vi "SCOPE Configuration_SA-Scope SP.vi"(6 "Timeout(10)":dbl=10.0, 7 "Operation":T1=enum."Initial", 8 "error in":errorcluster, 9 "Reset?(T)":bool=TRUE caption="reset device", 11 "Device. Name":string) -> (0 "error out":errorcluster, 1 "Status":string, 3 "InstruHandle":refnum<k15>, 4 "Rate":string, 5 "wfm":dbl[][](array[numeric]))   [LabVIEW 2012]
doc: "功能全局，处理对SCOPE的各种操作，包括：\n1.创建\n2.横向配置\n3.纵向配置\n4.触发配置\n5.关闭操作"
uses:
  <instrlib>/niScope/Controls/niScope vertical coupling.ctl
  <instrlib>/niScope/Controls/niScope self cal option.ctl
  Data Structure.llb/Function Variable Parameter Operations-Scope SP.ctl
  <instrlib>/niScope/Configure/Trigger/niScope Configure Trigger Window.vi
  <instrlib>/niScope/Configure/Trigger/niScope Configure Trigger Digital.vi
  <instrlib>/niScope/Configure/Trigger/niScope Configure Trigger Immediate.vi
  <instrlib>/niScope/Configure/Trigger/niScope Configure Trigger Hysteresis.vi
  <instrlib>/niScope/Configure/Trigger/niScope Configure Video Trigger.vi
  <instrlib>/niScope/Configure/Trigger/niScope Configure Trigger Edge.vi
  <instrlib>/niScope/Acquire/Fetch/niScope Multi Fetch.vi
  <instrlib>/niScope/Acquire/Fetch/niScope Fetch.vi
  <instrlib>/niScope/Configure/Trigger/niScope Configure Trigger Software.vi
  <instrlib>/NISCOPE/Controls/niScope scalar measurement.ctl
  SCOPE Operations_SA-Scope SP.ctl
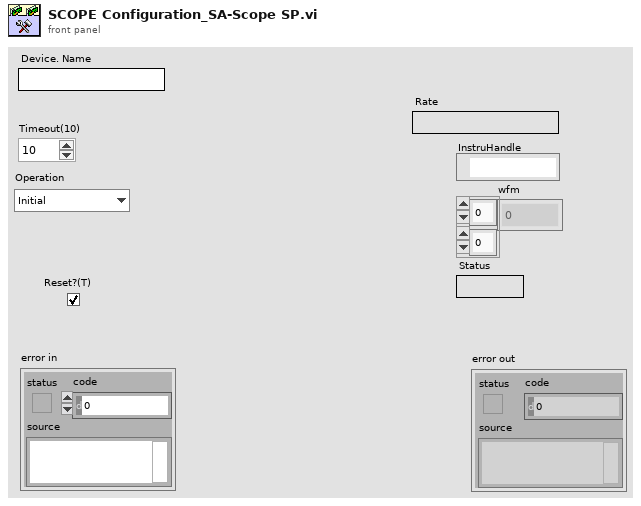
[diagram p1: front panel]
types:
  T1 = typedef "SCOPE Operations_SA-Scope SP.ctl" = enum16{"Noop", "Initial", "Horizontal", "Vertical", "Trigger", "RIS", "Initiate", "Fetch", "Abort", "Close", "SelfCalibrate", "AutoSetup"}
  T2 = typedef "Function Variable Parameter Operations-Scope SP.ctl" = enum16{"Set", "Get"}
  T3 = typedef "INI Initial Values_DStr-Scope SP.ctl" = cluster{"Active0":i32, "Acitive1":i32, "Channel":i32[], "ChanEnable":bool[], "ChanCpl":i32[], "OffsetVisible":bool[], "Offset":dbl[], "VoltInterval":i32[], "ProbAttenu":i32[], "Impedance":i32[], "BandWidth":i32[], "VertiPosi":dbl[], "Range":dbl[], "TimeInterval":i32, "Points":i32, "RefPosition":dbl, "Type":i32, "Source":i32, "TrigCpl":i32, "ExtCpl":i32, "Mode":i32, "Slope":i32, "Level":dbl, "Hyster":dbl, "WinMode":i32, "WinLow":dbl, "WinHigh":dbl, "Polarity":i32, "Event":i32, "Format":i32, "Line":i32, "DCRestore":bool, "RIS":bool, "Rate":dbl, "DigiSource":i32}
  T4 = typedef "INI Properties_DStr-Scope SP.ctl" = cluster{"Channels":cluster{"String":string, "Value":ext}[], "VoltInterval":cluster{"String":string, "Value":ext}[], "Impedance":cluster{"String":string, "Value":ext}[], "Bandwidth":cluster{"String":string, "Value":ext}[], "TimeInterval":cluster{"String":string, "Value":ext}[], "Type":cluster{"String":string, "Value":ext}[], "Source":cluster{"String":string, "Value":ext}[], "DigiSource":cluster{"String":string, "Value":ext}[], "TrigCpl":cluster{"String":string, "Value":ext}[], "EXTCpl":cluster{"String":string, "Value":ext}[], "Mode":cluster{"String":string, "Value":ext}[], "Event":cluster{"String":string, "Value":ext}[], "Format":cluster{"String":string, "Value":ext}[], "OffsetVisible":bool[], "Offset":dbl[][], "Point":dbl[][], "TrigLev":dbl[][], "Win":dbl[][], "Leve":dbl[][], "ExtLev":dbl[][], "PolaEnable":u8, "RISEnable":u8, "ChanCpl":cluster{"String":string, "Value":ext}[], "TimeValue":dbl[], "VoltValue":dbl[], "ImpedanceValue":dbl[], "BandwidthValue":dbl[]}
  T5 = typedef "niScope scalar measurement.ctl" = i32
  T6 = typedef "niScope vertical coupling.ctl" = i32
  T7 = cluster{"actualSamples":i32, "absoluteInitialX":dbl, "relativeInitialX":dbl, "xIncrement":dbl, "offset":dbl, "gain":dbl, "reserved1":dbl, "reserved2":dbl}
  T8 = cluster{"actualSamples":i32, "absoluteInitialX":dbl, "relativeInitialX":dbl, "xIncrement":dbl, "offset":dbl, "gain":dbl, "reserved1":dbl, "reserved2":dbl}[]
  T9 = typedef "niScope self cal option.ctl" = i32
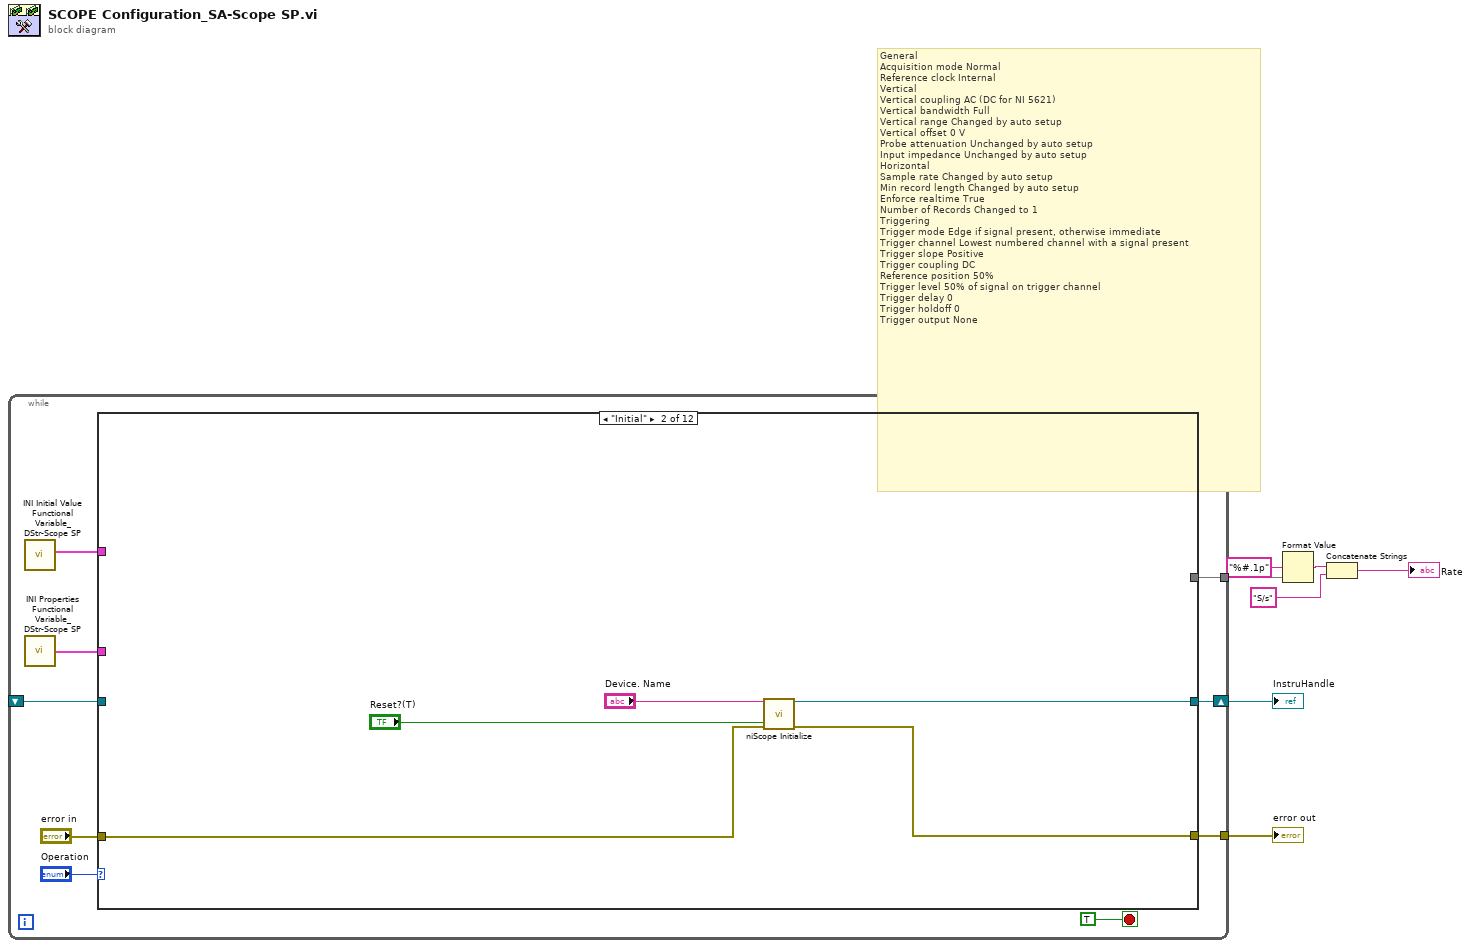
[diagram p0: block diagram]
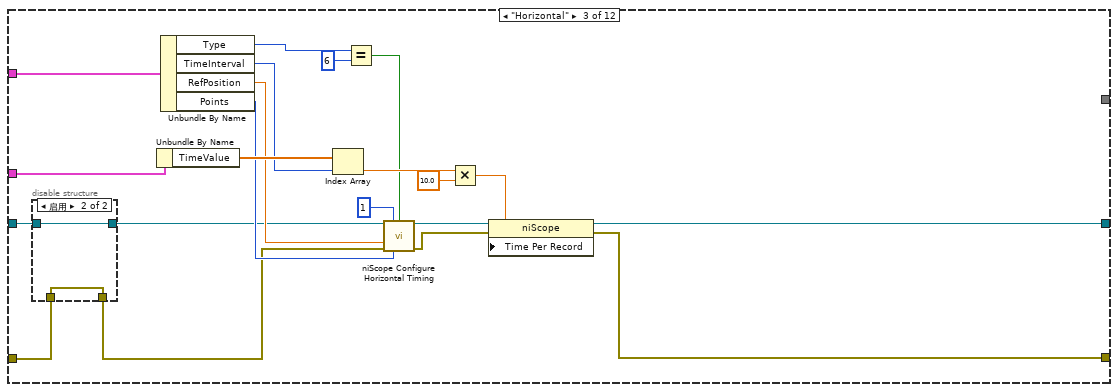
[diagram p3: hidden frame]
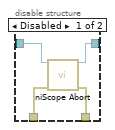
[diagram p4: hidden frame]
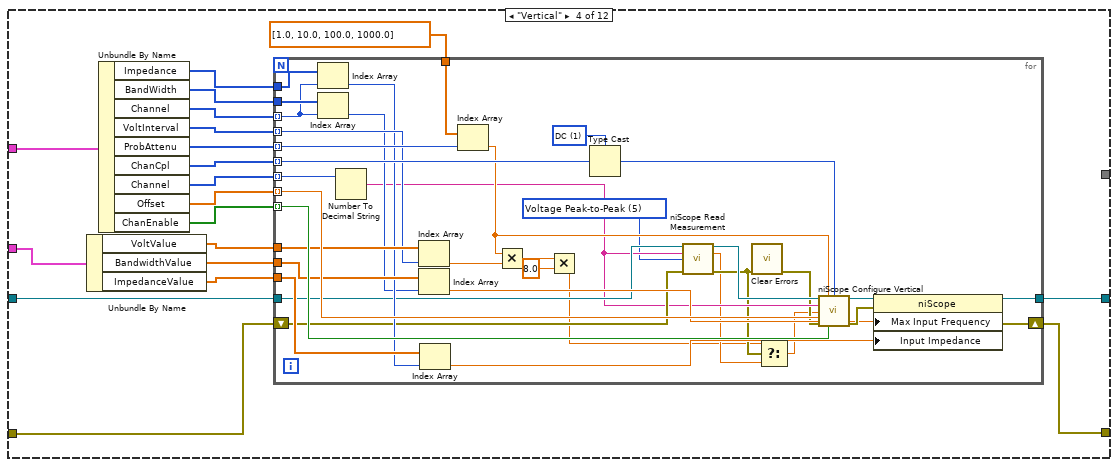
[diagram p5: hidden frame]
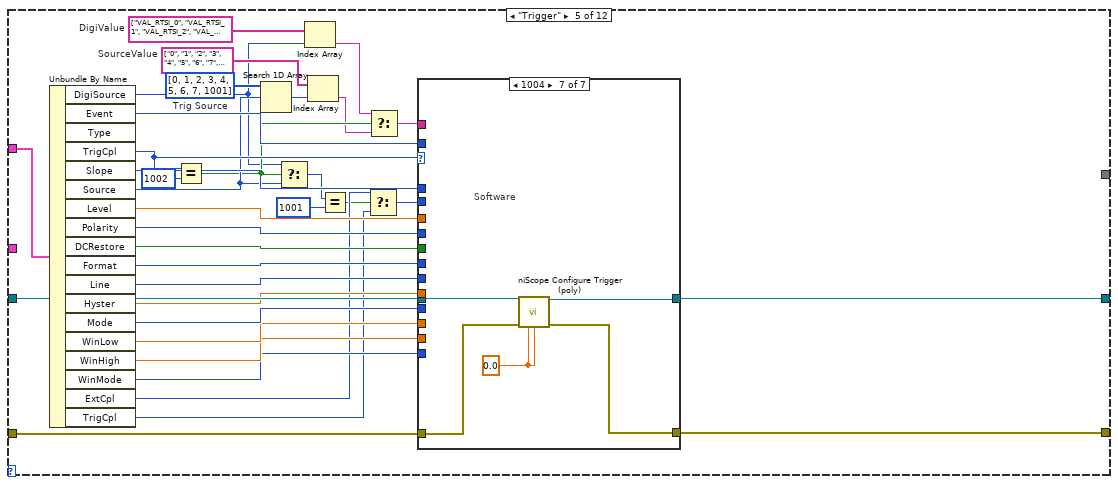
[diagram p6: hidden frame]
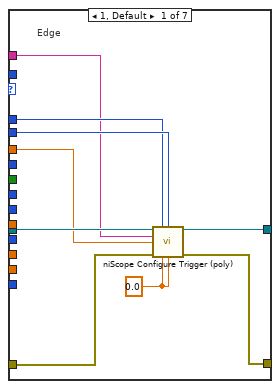
[diagram p7: hidden frame]
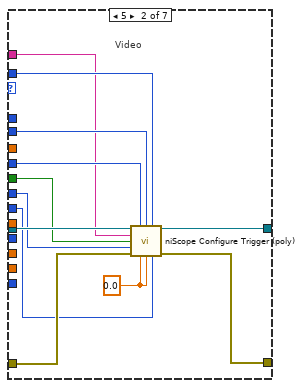
[diagram p8: hidden frame]
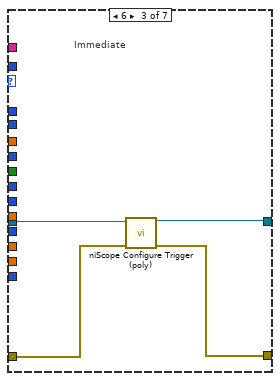
[diagram p9: hidden frame]
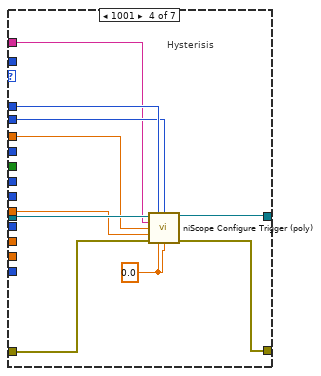
[diagram p10: hidden frame]
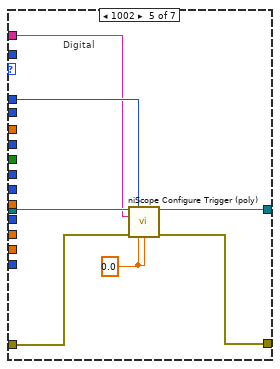
[diagram p11: hidden frame]
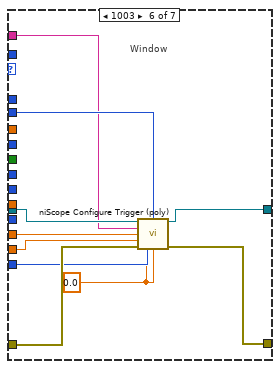
[diagram p12: hidden frame]
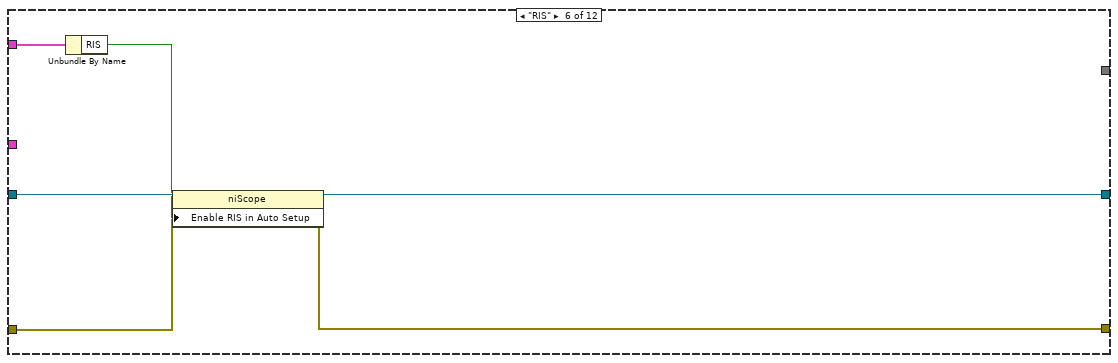
[diagram p13: hidden frame]
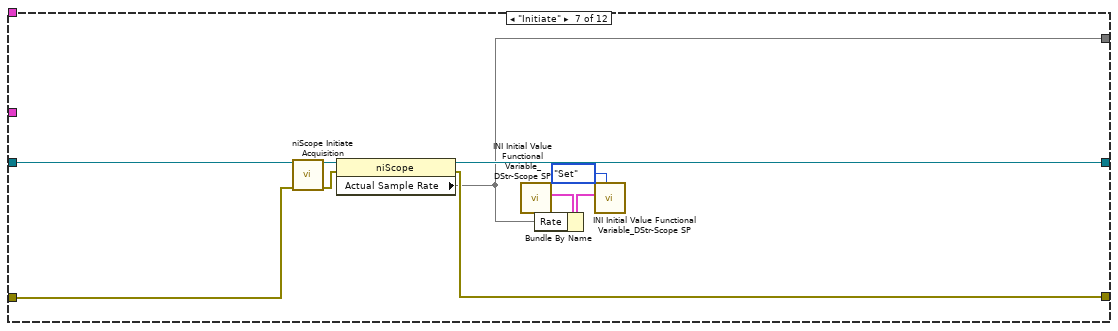
[diagram p14: hidden frame]
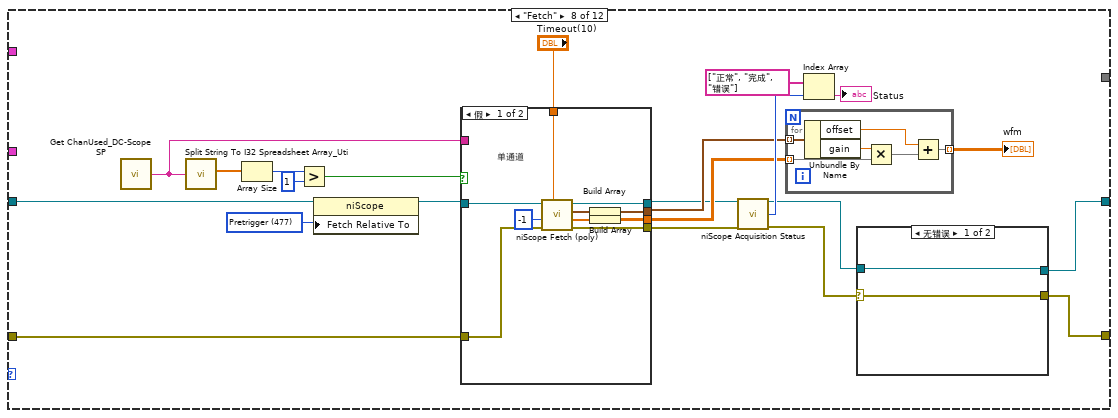
[diagram p15: hidden frame]
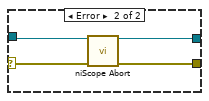
[diagram p16: hidden frame]
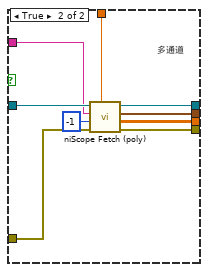
[diagram p17: hidden frame]
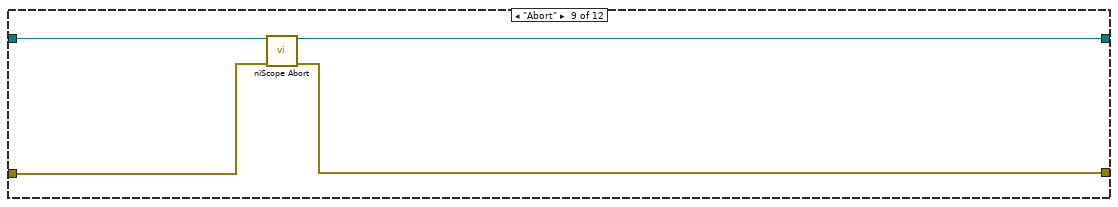
[diagram p18: hidden frame]
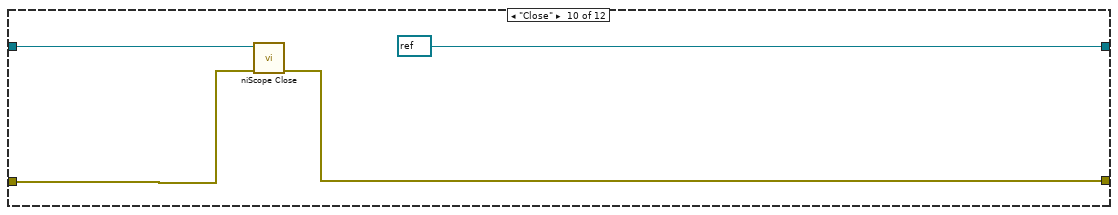
[diagram p19: hidden frame]
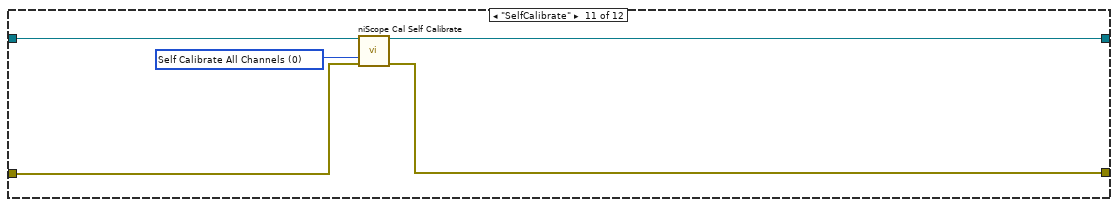
[diagram p20: hidden frame]
diagram:
  # "General \nAcquisition mode Normal  \nReference clock Internal  \nVertical \nVertical coupling AC (DC for NI 5621)  \nVertical bandwidth Full  \nVertical range Changed by auto setup  \nVertical offset 0 V  \nProbe attenuation Unchanged by auto setup  \nInput impedance Unchanged by auto setup  \nHorizontal \nSample rate Changed by auto setup  \nMin record length Changed by auto setup  \nEnforce realtime True  \nNumber of Records Changed to 1 \nTriggering \nTrigger mode Edge if signal present, otherwise immediate  \nTrigger channel Lowest numbered channel with a signal present  \nTrigger slope Positive  \nTrigger coupling DC  \nReference position 50%  \nTrigger level 50% of signal on trigger channel  \nTrigger delay 0  \nTrigger holdoff 0  \nTrigger output None"
  n1 = while {
    shift-right: [w14] -> w6
    shift-left: _ -> [w11]
    tunnel: [w12] -> w7
    tunnel: [w8] -> w2
    stop <- TRUE stop-if-true
    n2 = call "INI Initial Value Functional Variable_DStr-Scope SP.vi"() -> ("Value out"=w10:T3)  [unwired: 10 in, 1 out]
    n3 = call "INI Properties Functional Variable_DStr-Scope SP.vi"() -> ("proper"=w9:T4)  [unwired: 15 in]
    n4 = case shown="\"Initial\"" "Operation" {
      tunnel: [w18 w20 w41 w66 w139 w199 w209 w215 w268 refnum<k15> refnum ("instrument handle out") w277 w284] -> w14
      tunnel: "error in" -> [w17 w23 w27 w68 w141 w201 w213 w226 w270 w274 w279 w308]
      tunnel: [w17 w19 w38 w67 w140 w200 w208 w217 w269 w273 w278 w293] -> w12
      tunnel: w11 -> [w18 _ w26 w69 w138 w204 w214 w227 w271 w275 w280 w309]
      tunnel: w10 -> [_ _ w44 w65 w137 w203 _ _ _ _ _ w301]
      tunnel: w9 -> [_ _ w34 w58 _ _ _ _ _ _ _ w292]
      tunnel: [_ _ _ _ _ _ w207 _ _ _ _ w287] -> w8
      frame "Noop", Default {
      }
      frame "Initial" {
        n5 = call <instrlib>:"niScope Initialize.vi"("resource name"="Device. Name", "reset device"="Reset?(T)", "error in"=w23) -> ("instrument handle"=w20:refnum<k15>, "error out"=w19:errorcluster)  [unwired: 11 in]
      }
      frame "Horizontal" {
        n6 = disable-structure shown="启用" {
          disable-tunnel: w27 -> [w48 w49]
          disable-tunnel: w26 -> [w47 w50]
          disable-tunnel: [w46 w50] -> w25
          disable-tunnel: [w45 w49] -> w24
          frame Disabled {
            n7 = call <instrlib>:"niScope Abort.vi"("instrument handle"=w47, "error in"=w48) -> ("instrument handle out"=w46:refnum<k15>, "error out"=w45:errorcluster)  [unwired: 12 in]
          }
          frame Enabled {
          }
        }
        n8 = Unbundle By Name(w34) -> ("TimeValue"=w40:dbl[])
        n9 = Unbundle By Name(w44) -> ("Type"=w33:i32, "TimeInterval"=w30:i32, "RefPosition"=w28:dbl, "Points"=w29:i32)
        n10 = Index Array(array=w40, index=w30) -> (element=w37:dbl)
        n11 = Equal?(x=w33, y=6) -> (x = y?=w31:bool)
        n12 = call <instrlib>:"niScope Configure Horizontal Timing.vi"("instrument handle"=w25, "number of records"=1 ("f"), "enforce realtime"=w31, "reference position"=w28, "error in"=w24, "min record length"=w29) -> ("instrument handle out"=w42:refnum<k15>, "error out"=w39:errorcluster)  [unwired: 8 in]
        n13 = Multiply(x=w37, y=10.0) -> (x*y=w35:dbl)
        n14 = property class="niScope"(reference=w42, error in=w39, "Time Per Record"=w35) -> (reference out=w41:refnum<k15>, error out=w38:errorcluster)
      }
      frame "Vertical" {
        n15 = Unbundle By Name(w58) -> ("VoltValue"=w57:dbl[], "BandwidthValue"=w55:dbl[], "ImpedanceValue"=w54:dbl[])
        n16 = Unbundle By Name(w65) -> ("Impedance"=w52:i32[], "BandWidth"=w51:i32[], "Channel"=w53:i32[], "VoltInterval"=w56:i32[], "ProbAttenu"=w64:i32[], "ChanCpl"=w62:i32[], "Channel"=w61:i32[], "Offset"=w60:dbl[], "ChanEnable"=w59:bool[])
        n17 = for {
          tunnel: w69 -> [w78]
          shift-right: [w91] -> w67
          shift-left: w68 -> [w79]
          tunnel: [w93] -> w66
          tunnel: w64 -> [w99] mode=indexing
          tunnel: dbl[] [1.0, 10.0, 100.0, 1000.0] -> [w104]
          tunnel: w62 -> [w100] mode=indexing
          tunnel: w61 -> [w103] mode=indexing
          tunnel: w60 -> [w102] mode=indexing
          tunnel: w59 -> [w101] mode=indexing
          tunnel: w57 -> [w98]
          tunnel: w56 -> [w88] mode=indexing
          tunnel: w55 -> [w90]
          tunnel: w54 -> [w89]
          tunnel: w53 -> [w82] mode=indexing
          tunnel: w52 -> [w84]
          tunnel: w51 -> [w83]
          w75 = T5 5 items=["None"=4000, "Frequency"=2, "Average Frequency"=1016, "FFT Frequency"=1008, "Period"=3, "Average Period"=1015, "Rise Time"=0, "Fall Time"=1, "Rising Slew Rate"=1010, "Falling Slew Rate"=1011, "Overshoot"=18, "Preshoot"=19, "Voltage RMS"=4, "Voltage Cycle RMS"=16, "AC Estimate"=1012, "FFT Amplitude"=1009, "Voltage Average"=10, "Voltage Cycle Average"=17, "DC Estimate"=1013, "Voltage Max"=6, "Voltage Min"=7, "Voltage Peak-to-Peak"=5, "Voltage High"=8, "Voltage Low"=9, "Voltage Amplitude"=15, "Voltage Top"=1007, "Voltage Base"=1006, "Voltage Base-to-Top"=1017, "Negative Width"=11, "Positive Width"=12, "Negative Duty Cycle"=13, "Positive Duty Cycle"=14, "Integral"=1005, "Area"=1003, "Cycle Area"=1004, "Time Delay"=1014, "Phase Delay"=1018, "Low Ref Volts"=1000, "Mid Ref Volts"=1001, "High Ref Volts"=1002, "Volt. Hist. Mean"=2000, "Volt. Hist. Stdev"=2001, "Volt. Hist. Median"=2003, "Volt. Hist. Mode"=2010, "Volt. Hist. Max"=2005, "Volt. Hist. Min"=2006, "Volt. Hist. Peak-to-Peak"=2002, "Volt. Hist. Mean + Stdev"=2007, "Volt. Hist. Mean + 2 Stdev"=2008, "Volt. Hist. Mean + 3 Stdev"=2009, "Volt. Hist. Hits"=2004, "Volt. Hist. New Hits"=2011, "Time Hist. Mean"=3000, "Time Hist. Stdev"=3001, "Time Hist. Median"=3003, "Time Hist. Mode"=3010, "Time Hist. Max"=3005, "Time Hist. Min"=3006, "Time Hist. Peak-to-Peak"=3002, "Time Hist. Mean + Stdev"=3007, "Time Hist. Mean + 2 Stdev"=3008, "Time Hist. Mean + 3 Stdev"=3009, "Time Hist. Hits"=3004, "Time Hist. New Hits"=3011] ("scalar measurement")
          w106 = T6 1 items=["AC", "DC", "Ground"] ("vertical coupling")
          n18 = Index Array(array=w84, index=w82) -> (element=w81:i32)
          n19 = Index Array(array=w83, index=w82) -> (element=w80:i32)
          n20 = Number To Decimal String(number=w103) -> (decimal integer string=w76:string)  [unwired: 1 in]
          n21 = Index Array(array=w98, index=w88) -> (element=w97:dbl)
          n22 = Index Array(array=w90, index=w80) -> (element=w87:dbl)
          n23 = Index Array(array=w89, index=w81) -> (element=w86:dbl)
          n24 = Index Array(array=w104, index=w99) -> (element=w96:dbl)
          n25 = Multiply(x=w96, y=w97) -> (x*y=w95:dbl)
          n26 = Multiply(x=w95, y=8.0) -> (x*y=w70:dbl)
          n27 = Type Cast(type=w106, x=w100) -> (*(type *) &x=w105:T6)
          n28 = call <instrlib>:"niScope Read Measurement.vi"("instrument handle"=w78, "channels"=w76, "scalar measurement"=w75, "error in"=w79) -> ("instrument handle out"=w77:refnum<k15>, "result"=w71:dbl, "error out"=w73:errorcluster)  [unwired: 9 in]
          n29 = call <vilib>:"Clear Errors.vi"("error in (no error)"=w73) -> ("error out"=w74:errorcluster)  [unwired: 6 in]
          n30 = Select(t=w70, s=w73, f=w71) -> (s? t:f=w72:dbl)
          n31 = call <instrlib>:"niScope Configure Vertical.vi"("instrument handle"=w77, "probe attenuation"=w96, "vertical coupling"=w105, "channels"=w76, "vertical range"=w72, "vertical offset"=w102, "error in"=w74, "channel enabled"=w101) -> ("instrument handle out"=w94:refnum<k15>, "error out"=w92:errorcluster)  [unwired: 6 in]
          n32 = property class="niScope"(reference=w94, error in=w92, "Max Input Frequency"=w87, "Input Impedance"=w86) -> (reference out=w93:refnum<k15>, error out=w91:errorcluster)
        }
      }
      frame "Trigger" {
        w110 = string[] ["VAL_RTSI_0", "VAL_RTSI_1", "VAL_RTSI_2", "VAL_RTSI_3", "VAL_RTSI_4", "VAL_RTSI_5", "VAL_RTSI_6", "VAL_PFI_0", "VAL_PFI_1", "VAL_PFI_2", "VAL_PXI_STAR"]  # DigiValue
        w116 = string[] ["0", "1", "2", "3", "4", "5", "6", "7", "VAL_EXTERNAL"]  # SourceValue
        w114 = i32[] [0, 1, 2, 3, 4, 5, 6, 7, 1001]  # Trig Source
        n33 = Unbundle By Name(w137) -> ("DigiSource"=w109:i32, "Event"=w134:i32, "Type"=w121:i32, "Slope"=w136:i32, "Source"=w113:i32, "Level"=w135:dbl, "Polarity"=w133:i32, "DCRestore"=w132:bool, "Format"=w131:i32, "Line"=w130:i32, "Hyster"=w129:dbl, "Mode"=w128:i32, "WinLow"=w127:dbl, "WinHigh"=w126:dbl, "WinMode"=w125:i32, "ExtCpl"=w124:i32, "TrigCpl"=w122:i32)  [unwired: 1 out]
        n34 = Equal?(x=w121, y=1002) -> (x = y?=w112:bool)
        n35 = Search 1D Array(1D array=w114, element=w113) -> (index of element=w115:i32)  [unwired: 1 in]
        n36 = Select(t=w109, s=w112, f=w113) -> (s? t:f=w119:i32)
        n37 = Index Array(array=w110, index=w109) -> (element=w108:string)
        n38 = Index Array(array=w116, index=w115) -> (element=w111:string)
        n39 = Equal?(x=w119, y=1001) -> (x = y?=w117:bool)
        n40 = Select(t=w124, s=w117, f=w122) -> (s? t:f=w123:i32)
        n41 = Select(t=w108, s=w112, f=w111) -> (s? t:f=w107:string)
        n42 = case shown="1004" w121 {
          tunnel: w138 -> [w150 w162 w166 w176 w183 w193 w198]
          tunnel: [w143 w160 w164 w174 w181 w191 w196] -> w139
          tunnel: w141 -> [w149 w161 w165 w175 w182 w192 w197]
          tunnel: [w142 w159 w163 w173 w180 w190 w195] -> w140
          tunnel: w123 -> [w147 w158 _ w170 _ w189 _]
          tunnel: w136 -> [w146 _ _ w172 w179 _ _]
          tunnel: w135 -> [w148 _ _ w171 _ _ _]
          tunnel: w134 -> [_ w157 _ _ _ _ _]
          tunnel: w133 -> [_ w156 _ _ _ _ _]
          tunnel: w107 -> [w144 w155 _ w169 w178 w188 _]
          tunnel: w132 -> [_ w154 _ _ _ _ _]
          tunnel: w131 -> [_ w153 _ _ _ _ _]
          tunnel: w130 -> [_ w151 _ _ _ _ _]
          tunnel: w129 -> [_ _ _ w168 _ _ _]
          tunnel: w128 -> [_ _ _ _ _ _ _]
          tunnel: w127 -> [_ _ _ _ _ w187 _]
          tunnel: w126 -> [_ _ _ _ _ w186 _]
          tunnel: w125 -> [_ _ _ _ _ w185 _]
          frame 1, Default {
            w145 = 0.0 ("trigger holdoff")
            # "Edge"
            n43 = call-poly <instrlib>:"niScope Configure Trigger (poly).vi"("instrument handle"=w150, "trigger slope"=w146, "trigger coupling"=w147, "trigger source"=w144, "trigger level"=w148, "error in"=w149, "trigger holdoff"=w145, "trigger delay"=w145) -> ("instrument handle out"=w143:refnum<k15>, "error out"=w142:errorcluster)  [unwired: 6 in]
          }
          frame 5 {
            w152 = 0.0 ("trigger holdoff")
            # "Video"
            n44 = call-poly <instrlib>:"niScope Configure Trigger (poly).vi"("instrument handle"=w162, "polarity"=w156, "trigger coupling"=w158, "TV event"=w157, "trigger source"=w155, "enable DC restore"=w154, "signal format"=w153, "error in"=w161, "trigger holdoff"=w152, "trigger delay"=w152, "line number"=w151) -> ("instrument handle out"=w160:refnum<k15>, "error out"=w159:errorcluster)  [unwired: 3 in]
          }
          frame 6 {
            # "Immediate"
            n45 = call-poly <instrlib>:"niScope Configure Trigger (poly).vi"("instrument handle"=w166, "error in"=w165) -> ("instrument handle out"=w164:refnum<k15>, "error out"=w163:errorcluster)  [unwired: 12 in]
          }
          frame 1001 {
            w167 = 0.0 ("trigger holdoff")
            # "Hysterisis"
            n46 = call-poly <instrlib>:"niScope Configure Trigger (poly).vi"("instrument handle"=w176, "trigger slope"=w172, "trigger coupling"=w170, "trigger source"=w169, "trigger level"=w171, "hysteresis"=w168, "error in"=w175, "trigger holdoff"=w167, "trigger delay"=w167) -> ("instrument handle out"=w174:refnum<k15>, "error out"=w173:errorcluster)  [unwired: 5 in]
          }
          frame 1002 {
            w177 = 0.0 ("trigger holdoff")
            # "Digital"
            n47 = call-poly <instrlib>:"niScope Configure Trigger (poly).vi"("instrument handle"=w183, "trigger slope"=w179, "trigger source"=w178, "error in"=w182, "trigger holdoff"=w177, "trigger delay"=w177) -> ("instrument handle out"=w181:refnum<k15>, "error out"=w180:errorcluster)  [unwired: 8 in]
          }
          frame 1003 {
            w184 = 0.0 ("trigger delay")
            # "Window"
            n48 = call-poly <instrlib>:"niScope Configure Trigger (poly).vi"("instrument handle"=w193, "trigger window mode"=w185, "trigger coupling"=w189, "trigger source"=w188, "low level"=w187, "high level"=w186, "error in"=w192, "trigger holdoff"=w184, "trigger delay"=w184) -> ("instrument handle out"=w191:refnum<k15>, "error out"=w190:errorcluster)  [unwired: 5 in]
          }
          frame 1004 {
            w194 = 0.0 ("trigger holdoff")
            # "Software"
            n49 = call-poly <instrlib>:"niScope Configure Trigger (poly).vi"("instrument handle"=w198, "error in"=w197, "trigger holdoff"=w194, "trigger delay"=w194) -> ("instrument handle out"=w196:refnum<k15>, "error out"=w195:errorcluster)  [unwired: 10 in]
          }
        }
      }
      frame "RIS" {
        n50 = Unbundle By Name(w203) -> ("RIS"=w202:bool)
        n51 = property class="niScope"(reference=w204, error in=w201, "Enable RIS in Auto Setup"=w202) -> (reference out=w199:refnum<k15>, error out=w200:errorcluster)
      }
      frame "Initiate" {
        n52 = call <instrlib>:"niScope Initiate Acquisition.vi"("instrument handle"=w214, "error in"=w213) -> ("instrument handle out"=w206:refnum<k15>, "error out"=w205:errorcluster)  [unwired: 12 in]
        n53 = property class="niScope"(reference=w206, error in=w205) -> (reference out=w209:refnum<k15>, error out=w208:errorcluster, "Actual Sample Rate"=w207)
        n54 = call "INI Initial Value Functional Variable_DStr-Scope SP.vi"() -> ("Value out"=w212:T3)  [unwired: 10 in, 1 out]
        n55 = Bundle By Name(cluster=w212, "Rate"=w207) -> (w211:T3)
        n56 = call "INI Initial Value Functional Variable_DStr-Scope SP.vi"("Mode(Get)"=Function_Variable_Parameter_Operations-Scope_SP."Set", "Value in"=w211) -> ()  [unwired: 8 in, 2 out]
      }
      frame "Fetch" {
        w221 = 477 items=["Start"=482, "Trigger"=483, "Pretrigger"=477, "Now"=481, "Read Pointer"=388] ("Fetch:Fetch Relative To")
        n57 = call "Get ChanUsed_DC-Scope SP.vi"() -> ("ChanUsed"=w219:string)  [unwired: 1 in]
        n58 = call "Split String To I32 Spreadsheet Array_Uti.vi"("StringIn"=w219) -> ("Array"=w236:dbl[])  [unwired: 8 in, 1 out]
        n59 = Array Size(array=w236) -> (size(s)=w235:i32)
        n60 = Greater?(x=w235, y=1) -> (0:w233:bool)
        n61 = property class="niScope"(reference=w227, "Fetch Relative To"=w221) -> (reference out=w222:refnum<k15>)  [unwired: 1 in, 1 out]
        n62 = case shown="假" w233 {
          tunnel: w222 -> [w258 w267]
          tunnel: w226 -> [w257 w266]
          tunnel: [w256 w265] -> w231
          tunnel: [w255 w264] -> w223
          tunnel: [w251 w261] -> w225
          tunnel: [w250 w262] -> w224
          tunnel: "Timeout(10)" -> [w252 w263]
          tunnel: w219 -> [_ w259]
          frame False {
            # "单通道"
            n63 = call-poly <instrlib>:"niScope Fetch (poly).vi"("timeout"=w252, "error in"=w257, "numSamples"=-1, "instrument handle"=w258) -> ("error out"=w256:errorcluster, "wfm"=w253:dbl[], "wfm info"=w254:T7, "instrument handle out"=w255:refnum<k15>)  [unwired: 4 in]
            n64 = Build Array(w254) -> (w251:T8)
            n65 = Build Array(w253) -> (w250:dbl[][])
          }
          frame True {
            # "多通道"
            n66 = call-poly <instrlib>:"niScope Fetch (poly).vi"("timeout"=w263, "error in"=w266, "numSamples"=-1, "channels"=w259, "instrument handle"=w267) -> ("error out"=w265:errorcluster, "wfm"=w262:dbl[][], "wfm info"=w261:T8, "instrument handle out"=w264:refnum<k15>)  [unwired: 3 in]
          }
        }
        n67 = call <instrlib>:"niScope Acquisition Status.vi"("instrument handle"=w223, "error in"=w231) -> ("instrument handle out"=w216:refnum<k15>, "acquisition status"=w228:i32, "error out"=w218:errorcluster)  [unwired: 11 in]
        n68 = for {
          tunnel: w225 -> [w248] mode=indexing
          tunnel: w224 -> [w246] mode=indexing
          tunnel: [w243] -> w220 mode=indexing
          n69 = Unbundle By Name(w248) -> ("offset"=w244:dbl, "gain"=w247:dbl)
          n70 = Multiply(x=w247, y=w246) -> (x*y=w245:dbl[])
          n71 = Add(x=w244, y=w245) -> (x+y=w243:dbl[])
        }
        "wfm" <- w220
        n72 = Index Array(array=string[] ["正常", "完成", "错误"], index=w228) -> (element=→"Status":string)
        n73 = case shown="无错误" w218 {
          selector: w218 -> [w238 w242]
          tunnel: [w238 w241] -> w217
          tunnel: w216 -> [w237 w240]
          tunnel: [w237 w239] -> w215
          frame No Error {
          }
          frame Error {
            n74 = call <instrlib>:"niScope Abort.vi"("instrument handle"=w240, "error in"=w242) -> ("instrument handle out"=w239:refnum<k15>, "error out"=w241:errorcluster)  [unwired: 12 in]
          }
        }
      }
      frame "Abort" {
        n75 = call <instrlib>:"niScope Abort.vi"("instrument handle"=w271, "error in"=w270) -> ("instrument handle out"=w268:refnum<k15>, "error out"=w269:errorcluster)  [unwired: 12 in]
      }
      frame "Close" {
        n76 = call <instrlib>:"niScope Close.vi"("instrument handle"=w275, "error in"=w274) -> ("error out"=w273:errorcluster)  [unwired: 13 in]
      }
      frame "SelfCalibrate" {
        w276 = T9 0 items=["Self Calibrate All Channels", "Restore External Calibration"] ("Option")
        n77 = call <instrlib>:"niScope Cal Self Calibrate.vi"("instrument handle"=w280, "Option"=w276, "error in"=w279) -> ("instrument handle out"=w277:refnum<k15>, "error out"=w278:errorcluster)  [unwired: 11 in]
      }
      frame "AutoSetup" {
        n78 = Unbundle By Name(w301) -> ("Channel"=w303:i32[], "VoltInterval"=w282:i32[])
        n79 = Unbundle By Name(w292) -> ("TimeValue"=w291:dbl[])
        n80 = call <instrlib>:"niScope Auto Setup.vi"("instrument handle"=w309, "error in"=w308) -> ("instrument handle out"=w307:refnum<k15>, "error out"=w304:errorcluster)  [unwired: 12 in]
        n81 = Number To Decimal String(number=w303) -> (decimal integer string=w302:string[])  [unwired: 1 in]
        n82 = for {
          tunnel: w307 -> [w331]
          tunnel: [w338] -> w306
          tunnel: [w337] -> w305
          tunnel: w304 -> [w336]
          tunnel: w302 -> [w323] mode=indexing
          tunnel: [w335] -> w299 mode=indexing
          tunnel: [w334] -> w298 mode=indexing
          tunnel: [0.0] -> w297 mode=indexing
          tunnel: [w332] -> w296 mode=indexing
          tunnel: w282 -> [w326] mode=indexing
          tunnel: [w324] -> w281 mode=indexing
          w330 = T5 5 items=["None"=4000, "Frequency"=2, "Average Frequency"=1016, "FFT Frequency"=1008, "Period"=3, "Average Period"=1015, "Rise Time"=0, "Fall Time"=1, "Rising Slew Rate"=1010, "Falling Slew Rate"=1011, "Overshoot"=18, "Preshoot"=19, "Voltage RMS"=4, "Voltage Cycle RMS"=16, "AC Estimate"=1012, "FFT Amplitude"=1009, "Voltage Average"=10, "Voltage Cycle Average"=17, "DC Estimate"=1013, "Voltage Max"=6, "Voltage Min"=7, "Voltage Peak-to-Peak"=5, "Voltage High"=8, "Voltage Low"=9, "Voltage Amplitude"=15, "Voltage Top"=1007, "Voltage Base"=1006, "Voltage Base-to-Top"=1017, "Negative Width"=11, "Positive Width"=12, "Negative Duty Cycle"=13, "Positive Duty Cycle"=14, "Integral"=1005, "Area"=1003, "Cycle Area"=1004, "Time Delay"=1014, "Phase Delay"=1018, "Low Ref Volts"=1000, "Mid Ref Volts"=1001, "High Ref Volts"=1002, "Volt. Hist. Mean"=2000, "Volt. Hist. Stdev"=2001, "Volt. Hist. Median"=2003, "Volt. Hist. Mode"=2010, "Volt. Hist. Max"=2005, "Volt. Hist. Min"=2006, "Volt. Hist. Peak-to-Peak"=2002, "Volt. Hist. Mean + Stdev"=2007, "Volt. Hist. Mean + 2 Stdev"=2008, "Volt. Hist. Mean + 3 Stdev"=2009, "Volt. Hist. Hits"=2004, "Volt. Hist. New Hits"=2011, "Time Hist. Mean"=3000, "Time Hist. Stdev"=3001, "Time Hist. Median"=3003, "Time Hist. Mode"=3010, "Time Hist. Max"=3005, "Time Hist. Min"=3006, "Time Hist. Peak-to-Peak"=3002, "Time Hist. Mean + Stdev"=3007, "Time Hist. Mean + 2 Stdev"=3008, "Time Hist. Mean + 3 Stdev"=3009, "Time Hist. Hits"=3004, "Time Hist. New Hits"=3011] ("scalar measurement")
          n83 = property class="niScope" props=["Active Channel", "Channel Enabled", "Vertical Coupling", "Max Input Frequency", "Vertical Offset"](reference=w331, error in=w336, "Active Channel"=w323) -> (reference out=w338:refnum<k15>, error out=w337:errorcluster, "Channel Enabled"=w335, "Vertical Coupling"=w334, "Max Input Frequency"=w333)  [unwired: 1 out]
          n84 = call <instrlib>:"niScope Read Measurement.vi"("instrument handle"=w331, "timeout"=5.0, "channels"=w323, "scalar measurement"=w330) -> ("result"=w329:dbl, "error out"=w327:errorcluster)  [unwired: 9 in, 1 out]
          n85 = call "Set the Volt Interval According to Range in Autosetup_FP-Scope SP.vi"("PP"=w329) -> ("VoltInterval"=w325:i32)  [unwired: 14 in]
          n86 = call "Set the Impedancel According to Range in Autosetup_FP-Scope SP.vi"("BandWidth"=w333) -> ("BandWidth"=w332:i32)  [unwired: 14 in]
          n87 = Select(t=w326, s=w327, f=w325) -> (s? t:f=w324:i32)
        }
        n88 = Bundle By Name(cluster=w301, "ChanEnable"=w299, "ChanCpl"=w298, "BandWidth"=w296, "Offset"=w297, "VoltInterval"=w281) -> (w300:T3)
        n89 = property class="niScope" props=["Min Sample Rate", "Min Number of Points", "Enforce Realtime", "Number of Records", "Trigger Type", "Trigger Slope", "Trigger Coupling", "Trigger Source", "Trigger Level", "Trigger Delay", "Trigger Holdoff", "Trigger Hysteresis", "Reference Position"](reference=w306, error in=w305) -> (reference out=w294:refnum<k15>, error out=w295:errorcluster, "Min Sample Rate"=w287, "Min Number of Points"=w286, "Trigger Type"=w318, "Trigger Slope"=w317, "Trigger Coupling"=w316, "Trigger Source"=w315, "Trigger Level"=w313, "Trigger Hysteresis"=w312, "Reference Position"=w311)  [unwired: 4 out]
        n90 = Decimal String To Number(string=w315) -> (number=w314:i32)  [unwired: 2 in, 1 out]
        n91 = call "Set the TimeInterval According to Range in Autosetup_FP-Scope SP.vi"("Rate"=w287, "Points"=w286) -> ("VoltInterval"=w290:i32)  [unwired: 13 in]
        n92 = Index Array(array=w291, index=w290) -> (element=w288:dbl)
        n93 = Bundle By Name(cluster=w300, "Active0"=0, "Acitive1"=1, "Rate"=w287, "TimeInterval"=w290, "Points"=w286, "Type"=w318, "Slope"=w317, "TrigCpl"=w316, "Source"=w314, "Level"=w313, "Hyster"=w312, "RefPosition"=w311) -> (w310:T3)
        n94 = Multiply(x=w288, y=10.0) -> (x*y=w285:dbl)
        n95 = Divide(x=w286, y=w285) -> ()  [unwired: 1 out]
        n96 = property class="niScope"(reference=w294, error in=w295, "Time Per Record"=w285, "Enforce Realtime"=FALSE ("Horizontal:Enforce Realtime")) -> (reference out=w284:refnum<k15>, error out=w293:errorcluster)
        n97 = call "INI Initial Value Functional Variable_DStr-Scope SP.vi"("Mode(Get)"=Function_Variable_Parameter_Operations-Scope_SP."Set", "Value in"=w310) -> ()  [unwired: 8 in, 2 out]
      }
    }
  }
  "error out" <- w7
  "InstruHandle" <- w6
  n98 = Format Value(format string="%#.1p", value (0)=w2) -> (output string=w4:string)  [unwired: 1 in]
  n99 = Concatenate Strings(w4, "S/s" ("format string")) -> (→"Rate":string)
